vi "Label AsUnicode.vi"(0 "Ctl Refnum":refnum<vi>, 5 "Caption.Interpret As Unicode":bool, 11 "error in":errorcluster) -> (4 "reference out":refnum<vi>, 15 "error out":errorcluster)   [LabVIEW 2017]
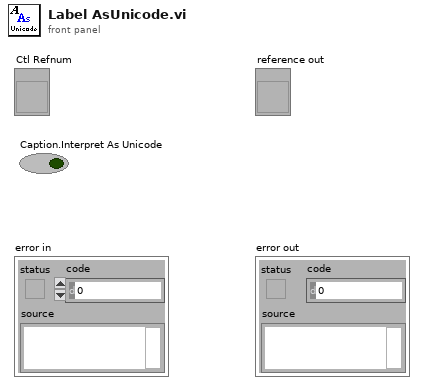
[diagram p1: front panel]
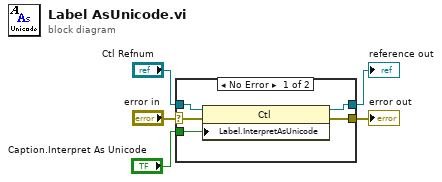
[diagram p0: block diagram]
diagram:
  n1 = case shown="No Error" "error in" {
    selector: "error in" -> [w8 w11]
    tunnel: "Ctl Refnum" -> [w10 w12]
    tunnel: "Caption.Interpret As Unicode" -> [w9 _]
    tunnel: [w7 w11] -> w3
    tunnel: [w6 w12] -> w2
    frame No Error {
      n2 = property class="Ctl"(reference=w10, error in=w8, "Label.InterpretAsUnicode"=w9) -> (reference out=w6:refnum<vi>, error out=w7:errorcluster)
    }
    frame Error {
    }
  }
  "error out" <- w3
  "reference out" <- w2
